vi "setUp.vi"(8 "error in":errorcluster, 11 "reference in":refnum<class "Examples.lvclass">) -> (0 "error out":errorcluster, 3 "reference out":refnum<class "Examples.lvclass">)   [LabVIEW 2020, in "Examples.lvclass"]
doc: "setUp runs prior to the test method during test execution. Use this method to initialize any object data required by your tests."
uses:
  Examples.lvclass
  C:/Program Files (x86)/National Instruments/LabVIEW 2020/vi.lib/addons/_JKI Toolkits/VI Tester/TestCase.llb/TestCase.lvclass
  Examples.lvclass/Examples.ctl
  <vilib>/addons/_JKI Toolkits/VI Tester/TestCase.llb/TestCase.lvclass
  niveristand-custom-device-testing-tools/VeriStandTestUtilities/VeriStandTestUtilities.lvlib
  C:/Git/niveristand-ballard-arinc429-custom-device/Source/Custom Device Support/Tests/System/Examples/Examples.lvclass
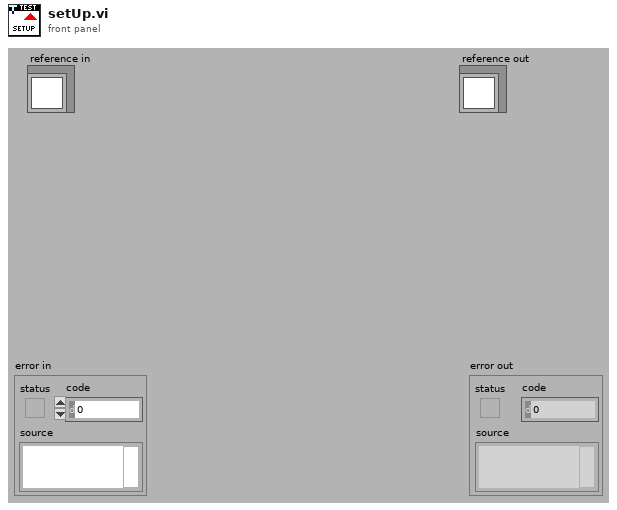
[diagram p1: front panel]
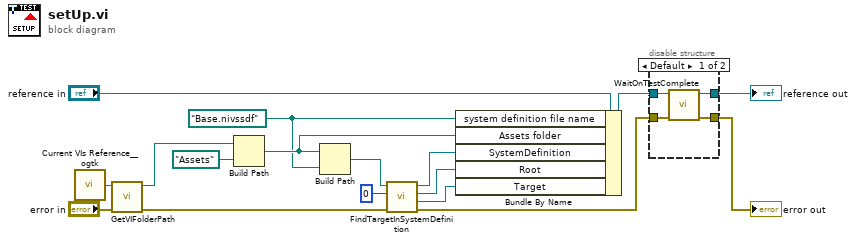
[diagram p0: block diagram]
diagram:
  w6 = path "Base.nivssdf" ("Absolute or Relative Path")
  n1 = call <userlib>:"Current VIs Reference__ogtk.vi"() -> ("Current VI's reference"=w15:refnum<vi>)  [unwired: 5 in]
  n2 = call "GetVIFolderPath.vi"("error in (no error)"="error in", "VI Reference in"=w15) -> ("error out"=w5:errorcluster, "VI Folder Path out"=w9:path)  [unwired: 8 in]
  n3 = Build Path(base path=w9, name or relative path=path "Assets" ("Absolute or Relative Path")) -> (appended path=w7:path)
  n4 = Build Path(base path=w7, name or relative path=w6) -> (appended path=w14:path)
  n5 = call "FindTargetInSystemDefinition.vi"("error in"=w5, "target index"=0 ("index"), "system definition path"=w14) -> ("error out"=w3:errorcluster, "Target"=w10:refnum<k24>, "Root"=w11:refnum<k24>, "System Definition"=w12:refnum<k24>)  [unwired: 5 in]
  n6 = Bundle By Name(cluster="reference in", "system definition file name"=w6, "Assets folder"=w7, "SystemDefinition"=w12, "Root"=w11, "Target"=w10) -> (w1:refnum<class "Examples.lvclass">)
  n7 = disable-structure shown="Default" {
    disable-tunnel: w3 -> [w21 w22]
    disable-tunnel: [w20 w22] -> w17
    disable-tunnel: [w19 w23] -> w16
    disable-tunnel: w1 -> [w18 w23]
    frame condition #0 (active) {
      n8 = call <vilib>:"WaitOnTestComplete.vi"("error in (no error)"=w21, "TestCase in"=w18) -> ("error out"=w20:errorcluster, "TestCase out"=w19:refnum<class "Examples.lvclass">)  [unwired: 8 in]
    }
    frame condition #1 {
    }
  }
  "error out" <- w17
  "reference out" <- w16
